vi "Report gen component (SubVI).vi"(11 "all rows":string[](array[string])) -> (3 "String":string)   [LabVIEW 2017]
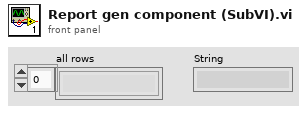
[diagram p1: front panel]
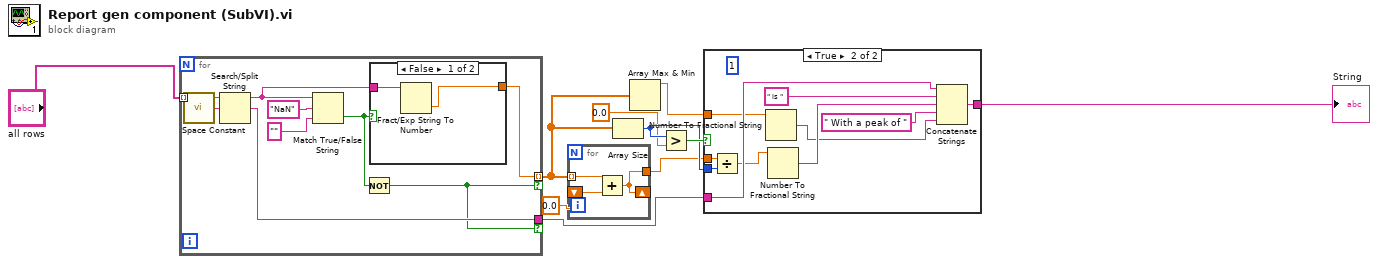
[diagram p0: block diagram]
diagram:
  n1 = for {
    tunnel: "all rows" -> [w19] mode=indexing
    tunnel: [w14] -> w3 mode=indexing if=w11
    tunnel: [w12] -> w4 if=w11
    n2 = call <vilib>:"Space Constant.vi"() -> ("String"=w18:string)
    n3 = Search/Split String(string=w19, search string/char (-)=w18) -> (substring before match=w15:string, match + rest of string=w12:string)  [unwired: 1 in, 1 out]
    n4 = Match True/False String(2:"" ("false string"), 3:"NaN" ("true string"), 4:w15) -> (0:w13:bool)  [unwired: 1 out]
    n5 = Not(x=w13) -> (.not. x?=w11:bool)
    n6 = case shown="False" w13 {
      tunnel: w15 -> [w21 _]
      tunnel: [w20 _] -> w14
      frame False {
        n7 = Fract/Exp String To Number(string=w21) -> (number=w20:dbl)  [unwired: 3 in, 1 out]
      }
      frame True {
      }
    }
  }
  n8 = for {
    shift-right: [w23] -> _
    shift-left: 0.0 -> [w24]
    tunnel: [w23] -> w2
    tunnel: w3 -> [w22] mode=indexing
    n9 = Add(x=w22, y=w24) -> (x+y=w23:dbl)
  }
  n10 = Array Size(array=w3) -> (size(s)=w8:i32)
  n11 = Array Max & Min(array=w3) -> (max value=w5:dbl)  [unwired: 3 out]
  n12 = Greater?(x=w8, y=0.0) -> (0:w9:bool)
  n13 = case shown="True" w9 {
    tunnel: w8 -> [_ w34]
    tunnel: w2 -> [_ w33]
    tunnel: w4 -> [_ w32]
    tunnel: w5 -> [_ w30]
    tunnel: [_ w29] -> w10
    frame False {
    }
    frame True {
      (unwired) 1
      n14 = Divide(x=w33, y=w34) -> (x/y=w31:dbl)
      n15 = Number To Fractional String(number=w30) -> (F-format string=w25:string)  [unwired: 3 in]
      n16 = Number To Fractional String(number=w31) -> (F-format string=w27:string)  [unwired: 3 in]
      n17 = Concatenate Strings(w32, " is ", w27, " With a peak of ", w25) -> (w29:string)
    }
  }
  "String" <- w10
